vi "Controller - Fire Command.vi"(8 "error in (no error)":errorcluster, 9 "Data":variant, 10 "CMD":T1=enum."Go Up", 11 "View Model":T2) -> (0 "error out":errorcluster, 3 "View Model":T2)   [LabVIEW 2017]
doc: "Fires Controller command User Event"
uses:
  View Model/Controls/View Model.ctl
  View Model/Controls/Shared Model.ctl
  Error Handler/Controls/Error Model.ctl
  Error Handler/Controls/Error Data.ctl
  Error Handler/Controls/Error Level.ctl
  Configuration/Controls/Config Model.ctl
  Configuration/Controls/Config Data Record.ctl
  Configuration/Controls/Config Command.ctl
  Controls/Control Model.ctl
  Controls/Elevator Location.ctl
  Controls/Elevator Status.ctl
  Controls/Control Event.ctl
  Controls/Control CMD.ctl
  Controls/Controller - Overhead.ctl
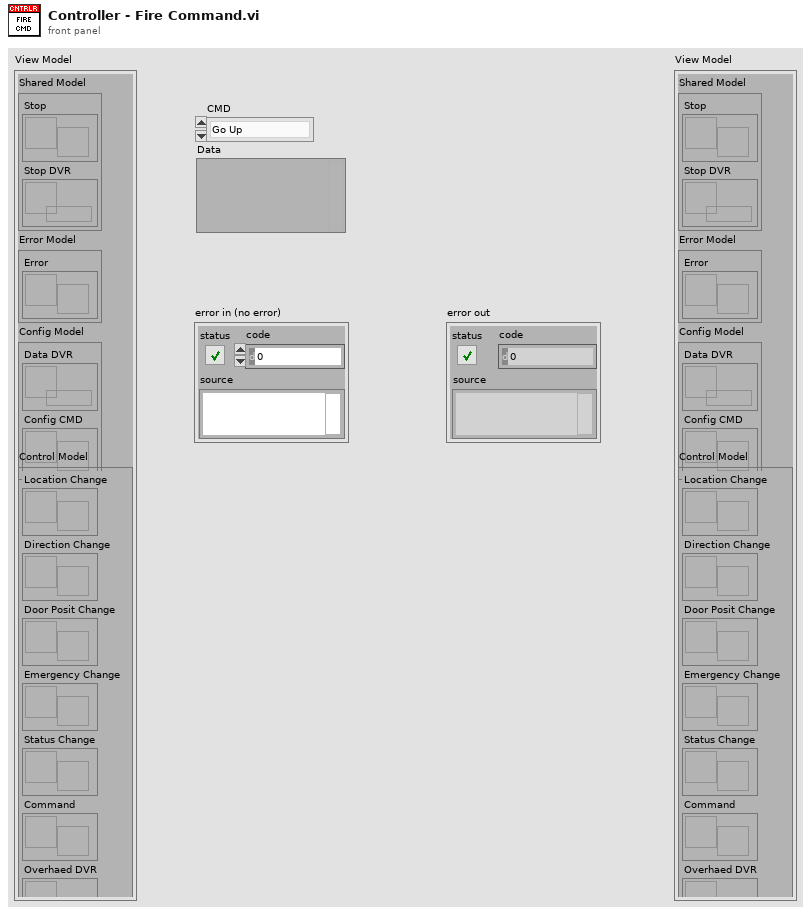
[diagram p1: front panel]
types:
  T1 = typedef "Control CMD.ctl" = enum16{"Idle", "Call", "Go Up", "Go Down", "Go to Floor", "Open Door", "Close Door", "Emergency"}
  T2 = typedef "View Model.ctl" = cluster{"Shared Model":T3, "Error Model":T4, "Config Model":T5, "Control Model":T6}
  T3 = typedef "Shared Model.ctl" = cluster{"Stop":refnum<user-event>, "Stop DVR":refnum<data-value>}
  T4 = typedef "Error Model.ctl" = cluster{"Error":refnum<user-event>}
  T5 = typedef "Config Model.ctl" = cluster{"Data DVR":refnum<data-value>, "Config CMD":refnum<user-event>}
  T6 = typedef "Control Model.ctl" = cluster{"Location Change":refnum<user-event>, "Direction Change":refnum<user-event>, "Door Posit Change":refnum<user-event>, "Emergency Change":refnum<user-event>, "Status Change":refnum<user-event>, "Command":refnum<user-event>, "Overhaed DVR":refnum<data-value>}
  T7 = typedef "Control Event.ctl" = cluster{"CMD":T1, "Data":variant}
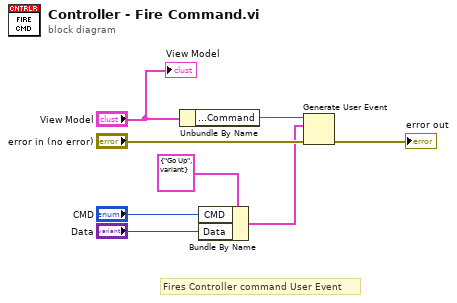
[diagram p0: block diagram]
diagram:
  # "Fires Controller command User Event"
  n1 = Unbundle By Name("View Model") -> ("Control Model.Command"=w8:refnum<user-event>)
  n2 = Bundle By Name(cluster=T7 {"CMD"=enum."Go Up", "Data"=variant} ("Controller Event"), "CMD"="CMD", "Data"="Data") -> (w1:T7)
  n3 = Generate User Event(user event=w8, event data cluster=w1, error in="error in (no error)") -> (error out=→"error out":errorcluster)  [unwired: 1 in, 1 out]
  "View Model" <- "View Model"
